vi "dilution walker.vi"() -> ()   [LabVIEW 2010]
uses:
  <userlib>/Nanonis Prog Interface V5/Nanonis Prog Interface.lvlib
panel:
  in  "Lockin offset (V)":dbl
  out "End":bool
  out "Pause":bool
  out "STM RX Temp":dbl
  in  "STM RX\nTemperature Limit (K)":dbl=7.0
  out "Mix Chamber Temp":dbl
  in  "Wait time (ms)":i32=2000
  in  "X Cap Upper limit (mV)":dbl=0.3
  in  "Current limit (nA)":dbl=10.0
  in  "X Cap Lower limit (mV)":dbl=0.2
  in  "Mixing Chamber\nTemperature Limit (K)":dbl=0.7
  in  "?":bool=TRUE
  in  "Number of Steps Increment":i32=100
  out "Z capacitance (pA)":cluster{"y":i32, sgl}[](graph)
  out "X capacitance (mV)":cluster{"y":i32, dbl}[](graph)
  in  "Lockin sensitivity (V)":dbl=0.02
  out "X capacitance (mV)":sgl
  out "Current (pA)":sgl
  out "Z capacitance (pA)":sgl
  # "+X"
  # "-X"
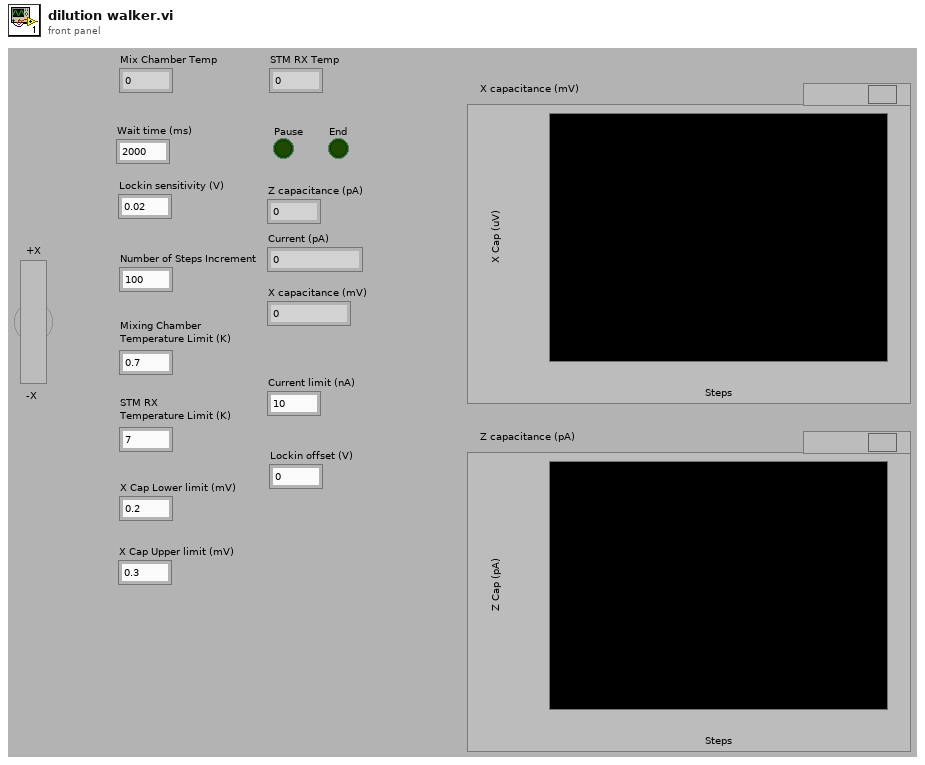
[diagram p1: front panel]
types:
  T1 = enum16{"Set Heater Voltage", "Read Heater Voltage", "Read Heater Current", "Read 1K Pot Temperature", "Read IVC Sorb Temperature", "Read Needle Valve Temperature", "Read Still Pressure", "Read Mixing Chamber Temperature", "Read STM RX Temperature", "Read STM CX Temperature", "Unstall Triton Loop", "Triton Stop", "Triton Stall Status"}
  T2 = enum8{"Group 1", "Group 2", "Group 3", "Group 4", "Group 5", "Group 6"}
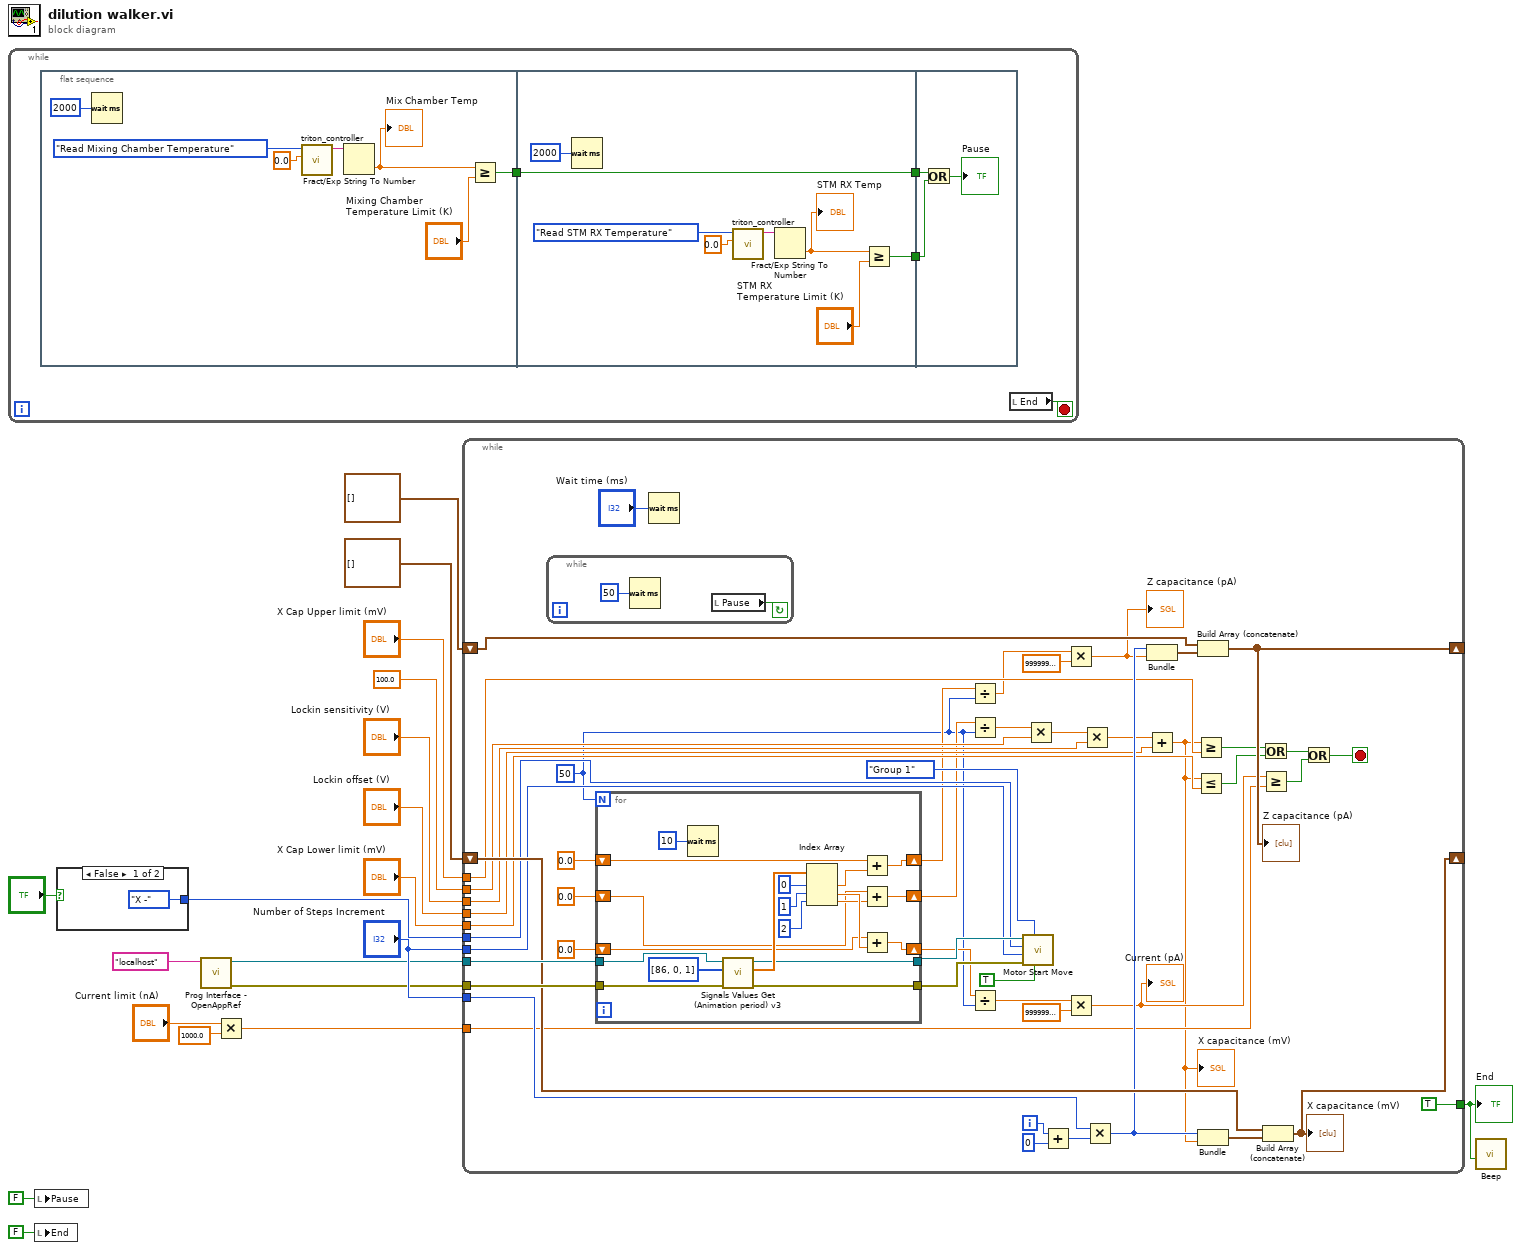
[diagram p0: block diagram]
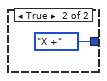
[diagram p2: hidden frame]
diagram:
  n1 = while {
    stop <- w20 stop-if-true
    n2 = flat-sequence {
      tunnel: [w24] -> w21
      tunnel: [w32] -> w23
      tunnel: [w31] -> w22
      tunnel: w21 -> [w31]
      tunnel: w23 -> [w41]
      tunnel: w22 -> [w40]
      frame #0 {
        n3 = Wait (ms)(milliseconds to wait=u32 2000) -> ()  [unwired: 1 out]
        n4 = call "triton_controller.vi"("Numerical Argument"=0.0, "Command"=T1."Read Mixing Chamber Temperature") -> ("Response"=w27:string)  [unwired: 9 in]
        n5 = Fract/Exp String To Number(string=w27) -> (number=w26:dbl)  [unwired: 3 in, 1 out]
        "Mix Chamber Temp" <- w26
        n6 = Greater Or Equal?(x=w26, y="Mixing Chamber\nTemperature Limit (K)") -> (x >= y?=w24:bool)
      }
      frame #1 {
        n7 = Wait (ms)(milliseconds to wait=u32 2000) -> ()  [unwired: 1 out]
        n8 = call "triton_controller.vi"("Numerical Argument"=0.0, "Command"=T1."Read STM RX Temperature") -> ("Response"=w35:string)  [unwired: 9 in]
        n9 = Fract/Exp String To Number(string=w35) -> (number=w33:dbl)  [unwired: 3 in, 1 out]
        "STM RX Temp" <- w33
        n10 = Greater Or Equal?(x=w33, y="STM RX\nTemperature Limit (K)") -> (x >= y?=w32:bool)
      }
      frame #2 {
        n11 = Or(x=w40, y=w41) -> (x .or. y?=→"Pause":bool)
      }
    }
    n12 = local read "End"() -> (w20:bool)
  }
  n13 = local write "Pause"(FALSE ("Pause")) -> ()
  n14 = local write "End"(FALSE ("End")) -> ()
  n15 = case shown="False" "?" {
    tunnel: [enum16{"X +", "X -", "Y +", "Y -", "Z +", "Z -"}."X -" ("Direction") enum16{"X +", "X -", "Y +", "Y -", "Z +", "Z -"}."X +" ("Direction")] -> w17
    frame False {
    }
    frame True {
    }
  }
  n16 = call <userlib>:"Prog Interface - OpenAppRef.vi"("Machine name (local machine IP)"="localhost" ("machine name (localhost)")) -> ("Error out"=w1:errorcluster, "Application reference"=w2:refnum<vi>)  [unwired: 5 in]
  n17 = Multiply(x="Current limit (nA)", y=1000.0) -> (x*y=w11:dbl)
  n18 = while {
    tunnel: w1 -> [w92]
    tunnel: w2 -> [w91]
    tunnel: "Lockin sensitivity (V)" -> [w66]
    tunnel: "Number of Steps Increment" -> [w86]
    shift-right: [w72] -> _
    shift-left: cluster{i32, sgl}[] [] -> [w84]
    shift-right: [w73] -> _
    shift-left: cluster{i32, sgl}[] [] -> [w81]
    tunnel: w17 -> [w77]
    tunnel: "Number of Steps Increment" -> [w76]
    tunnel: [TRUE] -> w15
    tunnel: 100.0 ("y") -> [w71]
    tunnel: w11 -> [w69]
    tunnel: "X Cap Upper limit (mV)" -> [w64]
    tunnel: "X Cap Lower limit (mV)" -> [w63]
    tunnel: "Lockin offset (V)" -> [w54]
    i -> [w67]
    stop <- w58 stop-if-true
    w44 = 50
    n19 = while {
      stop <- w113 continue-if-true
      n20 = Wait (ms)(milliseconds to wait=u32 50) -> ()  [unwired: 1 out]
      n21 = local read "Pause"() -> (w113:bool)
    }
    n22 = for {
      N: w44 -> [_]
      tunnel: w92 -> [w111]
      tunnel: w91 -> [w107]
      tunnel: [w104] -> w80
      tunnel: [w103] -> w79
      shift-right: [w100] -> w49
      shift-left: sgl 0.0 -> [w95]
      shift-right: [w99] -> w45
      shift-left: sgl 0.0 -> [w94]
      shift-right: [w96] -> w47
      shift-left: sgl 0.0 -> [w93]
      n23 = Wait (ms)(milliseconds to wait=u32 10) -> ()  [unwired: 1 out]
      n24 = call <userlib>:"Signals Values Get (Animation period) v3.vi"("error in (no error)"=w111, "Signals indexes (0-127)"=i8[] [86, 0, 1], "Application ref in"=w107) -> ("error out"=w103:errorcluster, "Signals Values"=w109:sgl[], "Application ref out"=w104:refnum<vi>)  [unwired: 5 in]
      n25 = Index Array(array=w109, index #1=0 ("index"), index #2=1 ("index"), index #3=2 ("index")) -> (element #1=w101:sgl, element #2=w98:sgl, element #3=w97:sgl)
      n26 = Add(x=w95, y=w101) -> (x+y=w100:sgl)
      n27 = Add(x=w93, y=w97) -> (x+y=w96:sgl)
      n28 = Add(x=w94, y=w98) -> (x+y=w99:sgl)
    }
    n29 = Wait (ms)(milliseconds to wait="Wait time (ms)") -> ()  [unwired: 1 out]
    n30 = Divide(x=w49, y=w44) -> (x/y=w50:sgl)
    n31 = Divide(x=w47, y=w44) -> (x/y=w48:sgl)
    n32 = Divide(x=w45, y=w44) -> (x/y=w46:sgl)
    n33 = call <userlib>:"Motor Start Move.vi"("Wait until finished? (F)"=TRUE, "Group"=T2."Group 1", "Error in (no error)"=w79, "Number of steps"=w76, "Direction"=w77, "Application ref in"=w80) -> ()  [unwired: 3 in, 2 out]
    n34 = Multiply(x=w48, y=w71) -> (x*y=w65:dbl)
    n35 = Add(x=w67, y=u16 0) -> (x+y=w87:i32)
    n36 = Multiply(x=w50, y=sgl 1000000000000.0) -> (x*y=w68:sgl)
    "Z capacitance (pA)" <- w68
    n37 = Multiply(x=w46, y=sgl 1000000000000.0) -> (x*y=w70:sgl)
    "Current (pA)" <- w70
    n38 = Multiply(x=w65, y=w66) -> (x*y=w55:dbl)
    n39 = Multiply(x=w86, y=w87) -> (x*y=w83:i32)
    n40 = Bundle(w83, w68) -> (w82:cluster{i32, sgl})  [unwired: 1 in]
    n41 = Add(x=w55, y=w54) -> (x+y=w56:dbl)
    "X capacitance (mV)" <- w56
    n42 = Greater Or Equal?(x=w56, y=w64) -> (x >= y?=w62:bool)
    n43 = Less Or Equal?(x=w56, y=w63) -> (x <= y?=w61:bool)
    n44 = Build Array (concatenate)(w81, w82) -> (w73:cluster{i32, sgl}[])
    "Z capacitance (pA)" <- w73
    n45 = Bundle(w83, w56) -> (w85:cluster{i32, dbl})  [unwired: 1 in]
    n46 = Or(x=w62, y=w61) -> (x .or. y?=w60:bool)
    n47 = Greater Or Equal?(x=w70, y=w69) -> (x >= y?=w59:bool)
    n48 = Build Array (concatenate)(w84, w85) -> (w72:cluster{i32, dbl}[])
    "X capacitance (mV)" <- w72
    n49 = Or(x=w60, y=w59) -> (x .or. y?=w58:bool)
  }
  "End" <- w15
  n50 = call <vilib>:"Beep.vi"("use system alert? (T)"=w15) -> ()  [unwired: 11 in]
